vi "ShooterStateController.vi"(1 "Selected State (In)":string) -> (0 "Selected State (Out)":string)   [LabVIEW 2019]
doc: "This VI makes all calculations and decisions related to the shooter subsystem."
uses:
  dsinstructions.vi
  sensors.vi
  constants.vi
  dsdata.vi
  outputs.vi
panel:
  in  "Shooter Prespin (ms)":u32=7000
  in  "Settling Time (ms)":u32=500
  in  "Shooter Off Delay (ms)":u32=1000
  in  "Max Range (in)":dbl=1000.0
  in  "Max Acceptable Robot Speed (ft/s)":dbl=5.0
  in  "Acceptable Shooter Error Fraction":dbl=0.1
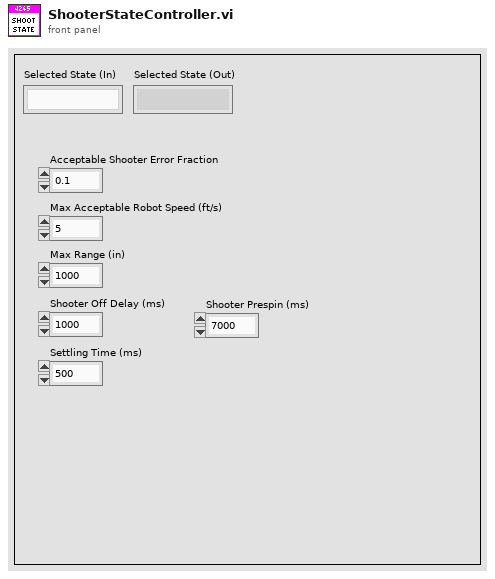
[diagram p1: front panel]
types:
  T1 = enum16{"Center", "North", "NorthWest", "West", "SouthWest", "South", "SouthEast", "East", "NorthEast"}
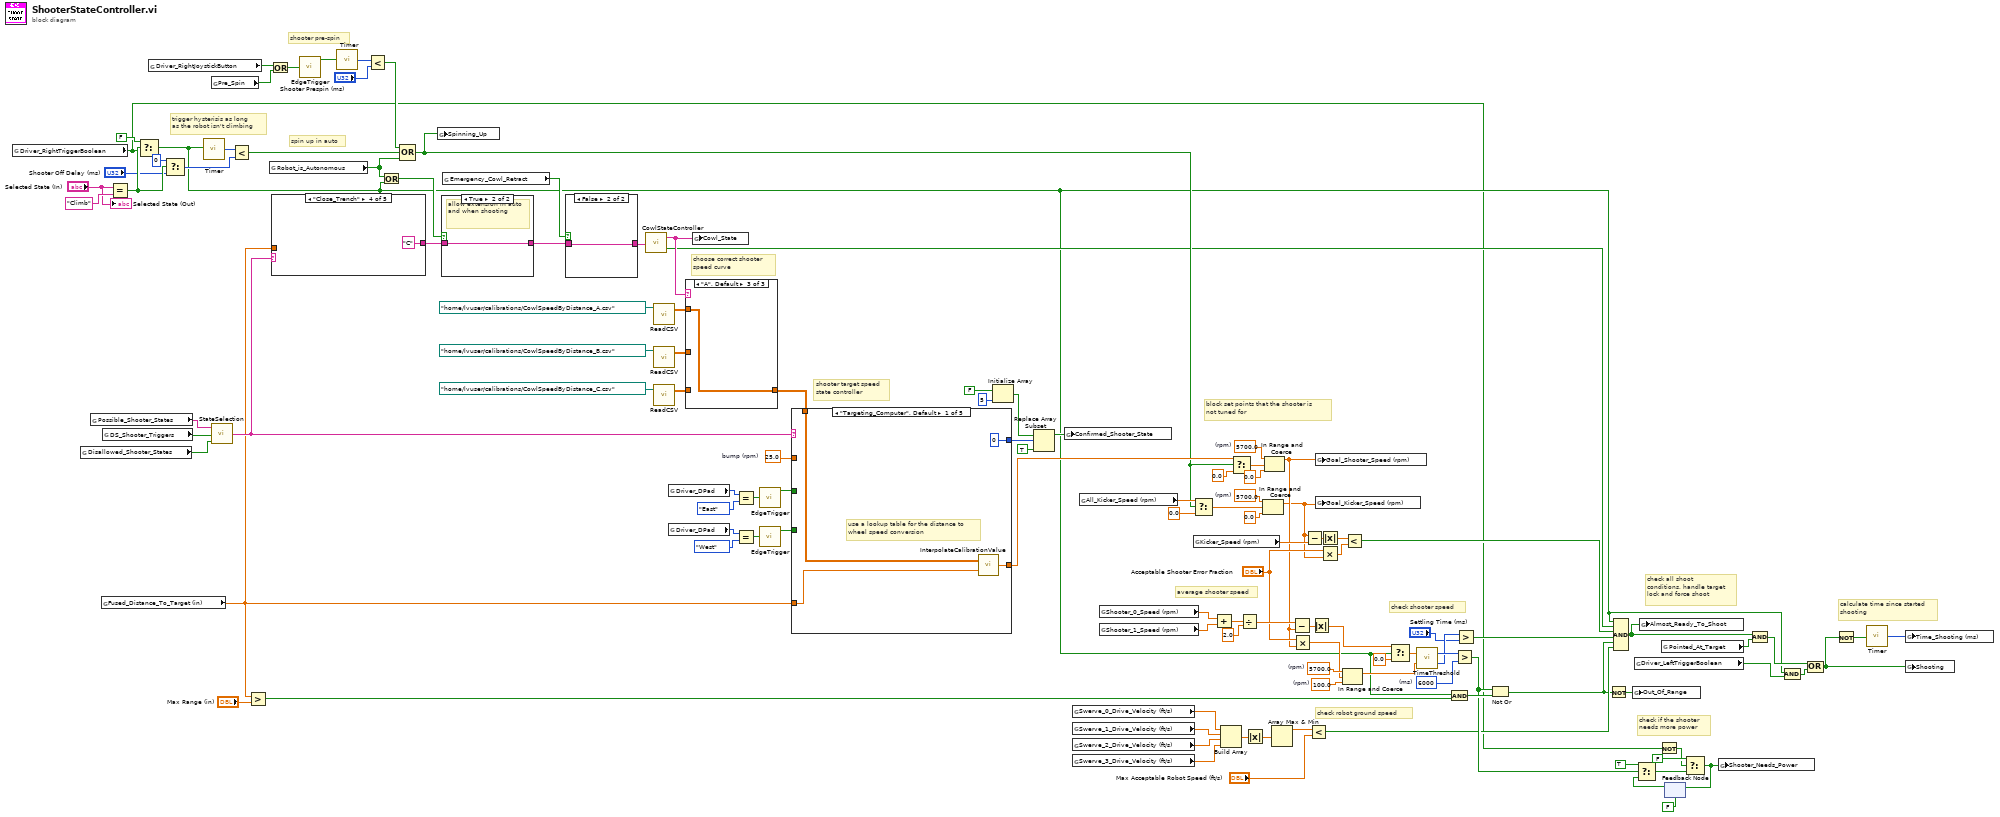
[diagram p0: block diagram]
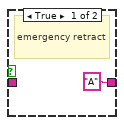
[diagram p2: hidden frame]
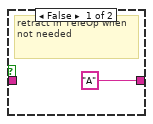
[diagram p3: hidden frame]
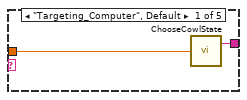
[diagram p4: hidden frame]
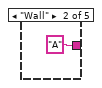
[diagram p5: hidden frame]
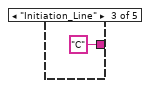
[diagram p6: hidden frame]
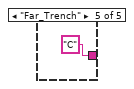
[diagram p7: hidden frame]
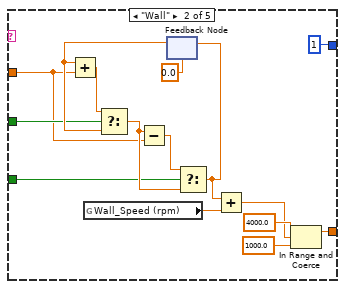
[diagram p10: hidden frame]
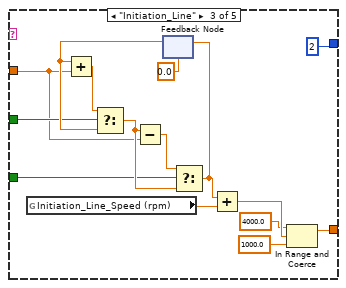
[diagram p11: hidden frame]
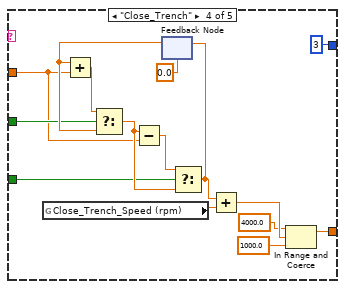
[diagram p12: hidden frame]
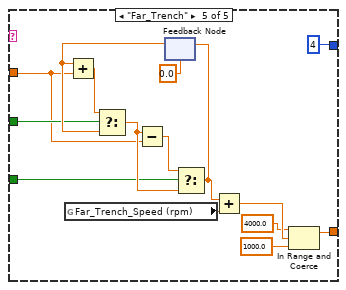
[diagram p13: hidden frame]
diagram:
  w8 = 25.0  # bump (rpm)
  w64 = 100.0  # (rpm)
  w65 = 5700.0  # (rpm)
  w73 = 5700.0  # (rpm)
  w77 = 5700.0  # (rpm)
  w92 = u32 6000  # (ms)
  # "calculate time since started\nshooting"
  # "check if the shooter\nneeds more power"
  # "average shooter speed"
  # "check shooter speed"
  # "shooter target speed\nstate controller"
  # "choose correct shooter\nspeed curve"
  # "shooter pre-spin"
  # "check all shoot\nconditions, handle target\nlock and force shoot"
  # "spin up in auto"
  # "trigger hysterisis as long\nas the robot isn't climbing"
  # "check robot ground speed"
  # "block set points that the shooter is \nnot tuned for"
  n1 = global read "dsinstructions.vi" "Driver_RightTriggerBoolean"() -> (w6:bool)
  n2 = global read "outputs.vi" "Disallowed_Shooter_States"() -> (w1:bool[])
  n3 = global read "constants.vi" "Possible_Shooter_States"() -> (w112:string[])
  n4 = global read "sensors.vi" "Fused_Distance_To_Target (in)"() -> (w79:dbl)
  n5 = global read "dsinstructions.vi" "DS_Shooter_Triggers"() -> (w111:bool[])
  n6 = Equal?(x="Selected State (In)", y="Climb") -> (x = y?=w51:bool)
  n7 = Select(t=FALSE, s=w51, f=w6) -> (s? t:f=w7:bool)
  n8 = global read "dsinstructions.vi" "Driver_RightJoystickButton"() -> (w24:bool)
  n9 = Select(t=u32 0, s=w51, f="Shooter Off Delay (ms)") -> (s? t:f=w48:u32)
  n10 = call "Timer.vi"("Reset Timer"=w7) -> ("Time (ms)"=w21:u32)
  n11 = global read "dsinstructions.vi" "Pre_Spin"() -> (w25:bool)
  n12 = call "StateSelection.vi"("Disallowed States"=w1, "State Triggers"=w111, "State Names"=w112) -> ("Selected State"=w85:string)
  n13 = Less?(x=w21, y=w48) -> (x < y?=w20:bool)
  n14 = Greater?(x=w79, y="Max Range (in)") -> (0:w56:bool)
  n15 = global read "dsdata.vi" "Robot_is_Autonomous"() -> (w2:bool)
  n16 = Or(x=w24, y=w25) -> (x .or. y?=w26:bool)
  n17 = case shown="\"Close_Trench\"" w85 {
    tunnel: w79 -> [w121 _ _ _ _]
    tunnel: [w122 "A" ("A,B,C") "C" ("A,B,C") "C" ("A,B,C") "C" ("A,B,C")] -> w84
    frame "Targeting_Computer", Default {
      n18 = call "ChooseCowlState.vi"("Distance (in)"=w121) -> ("Desired State"=w122:string)  [unwired: 1 in]
    }
    frame "Wall" {
    }
    frame "Initiation_Line" {
    }
    frame "Close_Trench" {
    }
    frame "Far_Trench" {
    }
  }
  n19 = call "EdgeTrigger.vi"("Input Signal"=w26) -> ("Rising Edge Trigger"=w23:bool)  [unwired: 2 out]
  n20 = call "Timer.vi"("Reset Timer"=w23) -> ("Time (ms)"=w22:u32)
  n21 = Less?(x=w22, y="Shooter Prespin (ms)") -> (x < y?=w35:bool)
  n22 = Or(x=w2, y=w7) -> (x .or. y?=w54:bool)
  n23 = Compound Arithmetic op=OR(w35, w20, w2) -> (w19:bool)
  n24 = global write "outputs.vi" "Spinning_Up"(w19) -> ()
  n25 = case shown="True" w54 {
    tunnel: w84 -> [_ w128]
    tunnel: ["A" ("A,B,C") w128] -> w83
    frame False {
      # "retract in TeleOp when not needed"
    }
    frame True {
      # "allow extension in auto and when shooting"
    }
  }
  n26 = global read "dsdata.vi" "Emergency_Cowl_Retract"() -> (w81:bool)
  n27 = case shown="False" w81 {
    tunnel: w83 -> [_ w130]
    tunnel: ["A" ("A,B,C") w130] -> w82
    frame True {
      # "emergency retract"
    }
    frame False {
    }
  }
  n28 = call "CowlStateController.vi"("Desired State"=w82) -> ("Current State"=w80:string, "Arrived"=w12:bool)
  n29 = call "ReadCSV.vi"("File Path (.csv)"=path "/home/lvuser/calibrations/CowlSpeedByDistance_A.csv" ("path")) -> ("Data (index by row)"=w89:dbl[][])  [unwired: 1 in, 1 out]
  n30 = call "ReadCSV.vi"("File Path (.csv)"=path "/home/lvuser/calibrations/CowlSpeedByDistance_B.csv" ("path")) -> ("Data (index by row)"=w88:dbl[][])  [unwired: 1 in, 1 out]
  n31 = call "ReadCSV.vi"("File Path (.csv)"=path "/home/lvuser/calibrations/CowlSpeedByDistance_C.csv" ("path")) -> ("Data (index by row)"=w87:dbl[][])  [unwired: 1 in, 1 out]
  n32 = global read "dsinstructions.vi" "Driver_DPad"() -> (w34:T1)
  n33 = global read "dsinstructions.vi" "Driver_DPad"() -> (w30:T1)
  n34 = case shown="\"A\", Default" w80 {
    tunnel: w89 -> [_ _ w133]
    tunnel: w88 -> [w131 _ _]
    tunnel: w87 -> [_ w132 _]
    tunnel: [w131 w132 w133] -> w86
    frame "B" {
    }
    frame "C" {
    }
    frame "A", Default {
    }
  }
  n35 = global write "outputs.vi" "Cowl_State"(w80) -> ()
  n36 = Equal?(x=w34, y=T1."East" ("Driver_DPad")) -> (x = y?=w32:bool)
  n37 = Equal?(x=w30, y=T1."West" ("Driver_DPad")) -> (x = y?=w29:bool)
  n38 = call "EdgeTrigger.vi"("Input Signal"=w32) -> ("Rising Edge Trigger"=w31:bool)  [unwired: 2 out]
  n39 = call "EdgeTrigger.vi"("Input Signal"=w29) -> ("Rising Edge Trigger"=w27:bool)  [unwired: 2 out]
  n40 = case shown="\"Targeting_Computer\", Default" w85 {
    tunnel: [w134 w147 w156 w171 w186] -> w110
    tunnel: [0 1 2 3 4] -> w104
    tunnel: w86 -> [w136 _ _ _ _]
    tunnel: w79 -> [w135 _ _ _ _]
    tunnel: w31 -> [_ w141 w154 w169 w184]
    tunnel: w27 -> [_ w140 w155 w170 w185]
    tunnel: w8 -> [_ w139 w153 w168 w183]
    frame "Targeting_Computer", Default {
      # "use a lookup table for the distance to\nwheel speed conversion"
      n41 = call "InterpolateCalibrationValue.vi"("Input"=w135, "Calibration Data"=w136) -> ("Interpolated Output"=w134:dbl)
    }
    frame "Wall" {
      n42 = global read "dsdata.vi" "Wall_Speed (rpm)"() -> (w143:dbl)
      n43 = feedback #1(0.0) -> (w145:dbl)
      n44 = Add(x=w145, y=w139) -> (x+y=w151:dbl)
      n45 = Select(t=w151, s=w141, f=w145) -> (s? t:f=w146:dbl)
      n46 = Subtract(x=w146, y=w139) -> (x-y=w148:dbl)
      n47 = Select(t=w148, s=w140, f=w146) -> (s? t:f=w138:dbl)
      n48 = feedback-in #1(w138) -> ()
      n49 = Add(x=w138, y=w143) -> (x+y=w142:dbl)
      n50 = In Range and Coerce(upper limit=4000.0, x=w142, lower limit=1000.0) -> (coerced(x)=w147:dbl)  [unwired: 1 out]
    }
    frame "Initiation_Line" {
      n51 = global read "dsdata.vi" "Initiation_Line_Speed (rpm)"() -> (w164:dbl)
      n52 = feedback #2(0.0) -> (w163:dbl)
      n53 = Add(x=w163, y=w153) -> (x+y=w160:dbl)
      n54 = Select(t=w160, s=w154, f=w163) -> (s? t:f=w162:dbl)
      n55 = Subtract(x=w162, y=w153) -> (x-y=w161:dbl)
      n56 = Select(t=w161, s=w155, f=w162) -> (s? t:f=w166:dbl)
      n57 = feedback-in #2(w166) -> ()
      n58 = Add(x=w166, y=w164) -> (x+y=w165:dbl)
      n59 = In Range and Coerce(upper limit=4000.0, x=w165, lower limit=1000.0) -> (coerced(x)=w156:dbl)  [unwired: 1 out]
    }
    frame "Close_Trench" {
      n60 = global read "dsdata.vi" "Close_Trench_Speed (rpm)"() -> (w179:dbl)
      n61 = feedback #3(0.0) -> (w178:dbl)
      n62 = Add(x=w178, y=w168) -> (x+y=w175:dbl)
      n63 = Select(t=w175, s=w169, f=w178) -> (s? t:f=w177:dbl)
      n64 = Subtract(x=w177, y=w168) -> (x-y=w176:dbl)
      n65 = Select(t=w176, s=w170, f=w177) -> (s? t:f=w181:dbl)
      n66 = feedback-in #3(w181) -> ()
      n67 = Add(x=w181, y=w179) -> (x+y=w180:dbl)
      n68 = In Range and Coerce(upper limit=4000.0, x=w180, lower limit=1000.0) -> (coerced(x)=w171:dbl)  [unwired: 1 out]
    }
    frame "Far_Trench" {
      n69 = global read "dsdata.vi" "Far_Trench_Speed (rpm)"() -> (w194:dbl)
      n70 = feedback #4(0.0) -> (w193:dbl)
      n71 = Add(x=w193, y=w183) -> (x+y=w190:dbl)
      n72 = Select(t=w190, s=w184, f=w193) -> (s? t:f=w192:dbl)
      n73 = Subtract(x=w192, y=w183) -> (x-y=w191:dbl)
      n74 = Select(t=w191, s=w185, f=w192) -> (s? t:f=w196:dbl)
      n75 = feedback-in #4(w196) -> ()
      n76 = Add(x=w196, y=w194) -> (x+y=w195:dbl)
      n77 = In Range and Coerce(upper limit=4000.0, x=w195, lower limit=1000.0) -> (coerced(x)=w186:dbl)  [unwired: 1 out]
    }
  }
  n78 = Initialize Array(FALSE, 5 ("dimension size")) -> (w107:bool[])
  n79 = Replace Array Subset(array=w107, new element=TRUE ("new element/subarray"), index=w104) -> (w105:bool[])
  n80 = global write "outputs.vi" "Confirmed_Shooter_State"(w105) -> ()
  n81 = global read "sensors.vi" "Swerve_0_Drive_Velocity (ft/s)"() -> (w102:dbl)
  n82 = global read "sensors.vi" "Swerve_1_Drive_Velocity (ft/s)"() -> (w101:dbl)
  n83 = global read "sensors.vi" "Swerve_2_Drive_Velocity (ft/s)"() -> (w100:dbl)
  n84 = global read "sensors.vi" "Swerve_3_Drive_Velocity (ft/s)"() -> (w99:dbl)
  n85 = global read "dsdata.vi" "All_Kicker_Speed (rpm)"() -> (w71:dbl)
  n86 = global read "sensors.vi" "Shooter_0_Speed (rpm)"() -> (w118:dbl)
  n87 = global read "sensors.vi" "Shooter_1_Speed (rpm)"() -> (w117:dbl)
  n88 = Select(t=w71, s=w19, f=0.0) -> (s? t:f=w70:dbl)
  n89 = global read "sensors.vi" "Kicker_Speed (rpm)"() -> (w69:dbl)
  n90 = Add(x=w118, y=w117) -> (x+y=w116:dbl)
  n91 = Build Array(w102, w101, w100, w99) -> (w98:dbl[])
  n92 = Select(t=w110, s=w19, f=0.0) -> (s? t:f=w78:dbl)
  n93 = Divide(x=w116, y=2.0) -> (x/y=w113:dbl)
  n94 = Absolute Value(x=w98) -> (abs(x)=w97:dbl[])
  n95 = In Range and Coerce(upper limit=w73, x=w70, lower limit=0.0) -> (coerced(x)=w18:dbl)  [unwired: 1 out]
  n96 = In Range and Coerce(upper limit=w77, x=w78, lower limit=0.0) -> (coerced(x)=w60:dbl)  [unwired: 1 out]
  n97 = Array Max & Min(array=w97) -> (max value=w96:dbl)  [unwired: 3 out]
  n98 = Subtract(x=w113, y=w60) -> (x-y=w114:dbl)
  n99 = Multiply(x="Acceptable Shooter Error Fraction", y=w60) -> (x*y=w63:dbl)
  n100 = Subtract(x=w18, y=w69) -> (x-y=w68:dbl)
  n101 = Less?(x=w96, y="Max Acceptable Robot Speed (ft/s)") -> (x < y?=w17:bool)
  n102 = Absolute Value(x=w114) -> (abs(x)=w59:dbl)
  n103 = global write "outputs.vi" "Goal_Shooter_Speed (rpm)"(w60) -> ()
  n104 = global write "outputs.vi" "Goal_Kicker_Speed (rpm)"(w18) -> ()
  n105 = Absolute Value(x=w68) -> (abs(x)=w61:dbl)
  n106 = Multiply(x="Acceptable Shooter Error Fraction", y=w18) -> (x*y=w66:dbl)
  n107 = In Range and Coerce(upper limit=w65, x=w63, lower limit=w64) -> (coerced(x)=w62:dbl)  [unwired: 1 out]
  n108 = Less?(x=w61, y=w66) -> (x < y?=w13:bool)
  n109 = Select(t=w59, s=w7, f=0.0) -> (s? t:f=w58:dbl)
  n110 = call "TimeThreshold.vi"("Threshold"=w62, "Current Value"=w58) -> ("Time Below Threshold (ms)"=w38:u32, "Time Above Threshold (ms)"=w93:u32)
  n111 = And(x=w7, y=w56) -> (x .and. y?=w55:bool)
  n112 = Greater?(x=w93, y=w92) -> (0:w46:bool)
  n113 = Greater?(x=w38, y="Settling Time (ms)") -> (0:w14:bool)
  n114 = Not Or(1:w55, 2:w46) -> (0:w15:bool)
  n115 = Not(x=w15) -> (.not. x?=w16:bool)
  n116 = Compound Arithmetic op=AND(w7, w12, w13, w14, w15, w17) -> (w11:bool)
  n117 = global write "outputs.vi" "Out_Of_Range"(w16) -> ()
  n118 = global read "dsinstructions.vi" "Driver_LeftTriggerBoolean"() -> (w10:bool)
  n119 = global write "outputs.vi" "Almost_Ready_To_Shoot"(w11) -> ()
  n120 = Not(x=w6) -> (.not. x?=w39:bool)
  n121 = global read "sensors.vi" "Pointed_At_Target"() -> (w75:bool)
  n122 = feedback #5(FALSE) -> (w44:bool)
  n123 = Select(t=TRUE, s=w46, f=w44) -> (s? t:f=w42:bool)
  n124 = Select(t=FALSE, s=w39, f=w42) -> (s? t:f=w40:bool)
  n125 = feedback-in #5(w40) -> ()
  n126 = global write "outputs.vi" "Shooter_Needs_Power"(w40) -> ()
  n127 = Compound Arithmetic op=AND(w11, w75) -> (w76:bool)
  n128 = Compound Arithmetic op=AND(w7, w10) -> (w9:bool)
  n129 = Compound Arithmetic op=OR(w76, w9) -> (w5:bool)
  n130 = Not(x=w5) -> (.not. x?=w4:bool)
  n131 = call "Timer.vi"("Reset Timer"=w4) -> ("Time (ms)"=w3:u32)
  n132 = global write "outputs.vi" "Time_Shooting (ms)"(w3) -> ()
  n133 = global write "outputs.vi" "Shooting"(w5) -> ()
  "Selected State (Out)" <- "Selected State (In)"
